vi "NI save one frame AI data.vi"(8 "error in (no error)":errorcluster, 10 "file path":path, 11 "NI in":refnum<class "NI.lvclass">) -> (0 "error out":errorcluster, 3 "NI out":refnum<class "NI.lvclass">)   [LabVIEW 2021, in "NI.lvlib" / "NI.lvclass"]
uses:
  NI.lvclass
  NI.lvclass/NI.ctl
  <vilib>/DAQmx/read.llb/DAQmx Read (Analog 1D DBL 1Chan NSamp).vi
  <vilib>/DAQmx/miscellaneous.llb/DAQmx Fill In Error Info.vi
  <vilib>/Utility/file.llb/Write Delimited Spreadsheet (DBL).vi
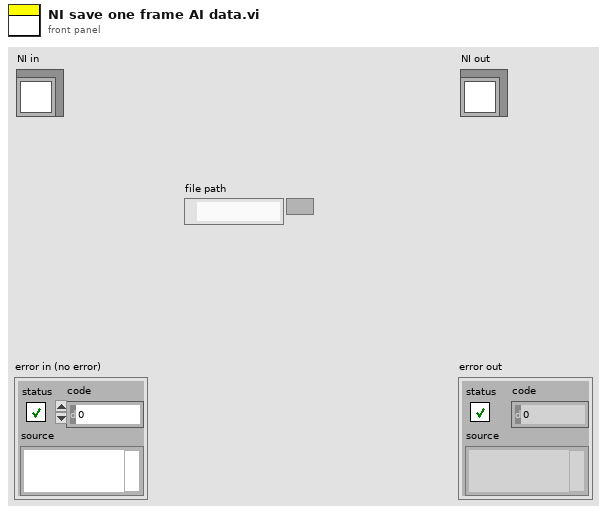
[diagram p1: front panel]
types:
  T1 = typedef "NI.lvlib/NI.lvclass/NI task parameters.ctl" = cluster{"exposure time":dbl, "camera H":dbl, "y line #":dbl, "flyback line #":dbl, "y pixel size":dbl, "z scan #":dbl, "z step size":dbl, "z offset":dbl, "laser all on?":bool, "laser option":bool[]}
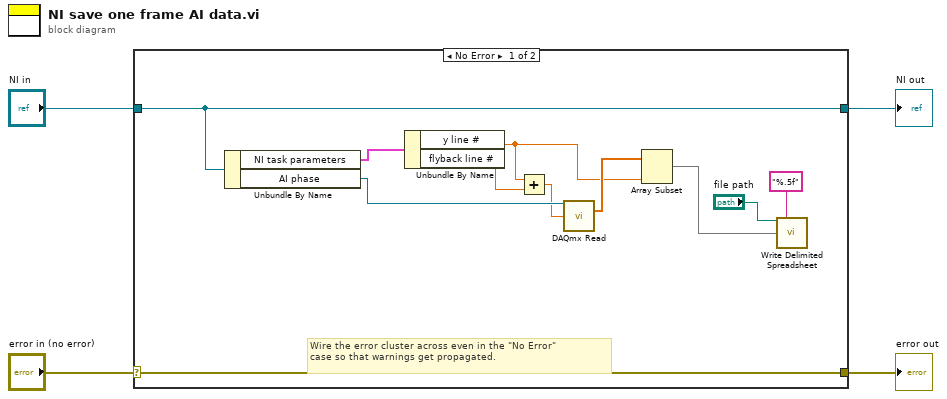
[diagram p0: block diagram]
diagram:
  n1 = case shown="No Error" "error in (no error)" {
    selector: "error in (no error)" -> [w15 w17]
    tunnel: [w15 w17] -> w3
    tunnel: [w14 w16] -> w1
    tunnel: "NI in" -> [w14 w16]
    frame No Error {
      # "Wire the error cluster across even in the \"No Error\"\ncase so that warnings get propagated."
      n2 = Unbundle By Name(w14) -> ("NI task parameters"=w13:T1, "AI phase"=w12:refnum<k21>)
      n3 = Unbundle By Name(w13) -> ("y line #"=w8:dbl, "flyback line #"=w11:dbl)
      n4 = Add(x=w8, y=w11) -> (x+y=w10:dbl)
      n5 = call-poly <vilib>:"DAQmx Read.vi"("task/channels in"=w12, "number of samples per channel"=w10) -> ("data"=w9:dbl[])  [unwired: 11 in, 2 out]
      n6 = Array Subset(array=w9, length=w8) -> (w6:dbl[])  [unwired: 1 in]
      n7 = call-poly <vilib>:"Write Delimited Spreadsheet.vi"("file path (dialog if empty)"="file path", "format (%.3f)"="%.5f", "1D data"=w6) -> ()  [unwired: 11 in, 2 out]
    }
    frame Error {
    }
  }
  "error out" <- w3
  "NI out" <- w1
